vi "Configure IQ Input.vi"(6 "Voltage Level (0.4 V)":dbl=0.4, 7 "I/Q Input Level Method (0: Default)":i32(ring) items=["Default", "Manual", "Measurement"], 8 "error in (no error)":errorcluster, 9 "Auto Attenuation (T: Enable)":bool=TRUE, 10 "Attenuation Level (2 dB)":dbl=2.0, 11 "VISA resource name":refnum<visa-resource-name>) -> (0 "error out":errorcluster, 3 "VISA resource name out":refnum<visa-resource-name>)   [LabVIEW 2012, in "Agilent PSG MXG Series.lvlib"]
doc: "Configures attenuation mode, attenuation level, external I/Q input level and method.\n\n<B>Notes:</B>\n(1) This VI is valid only in N5172B and N5182B."
uses:
  <instrlib>/Agilent PSG MXG Series/Agilent PSG MXG Series.lvlib
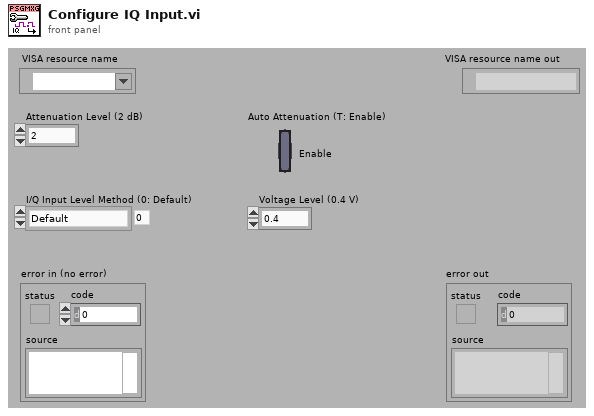
[diagram p1: front panel]
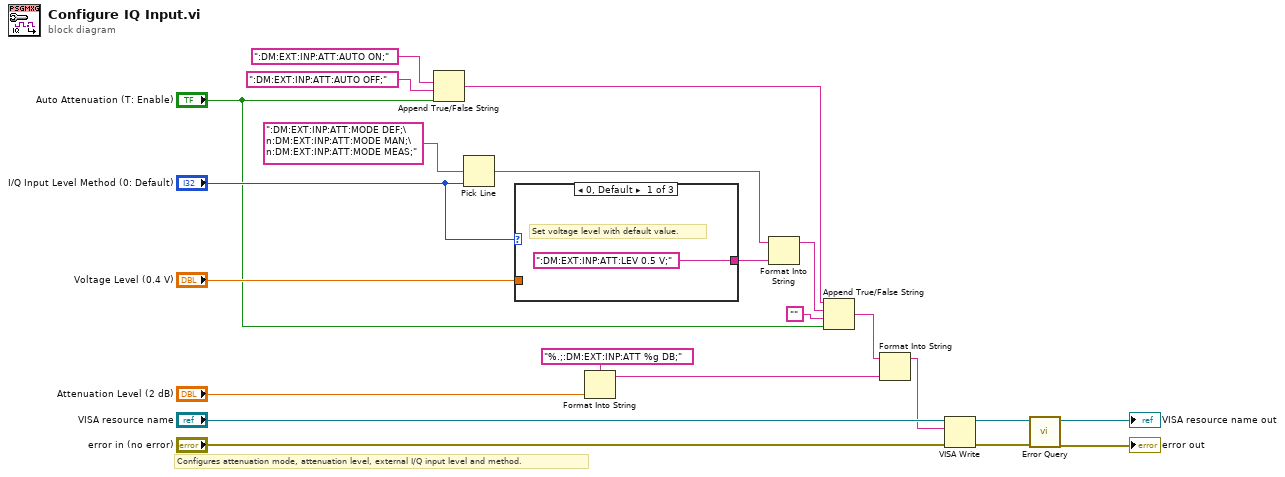
[diagram p0: block diagram]
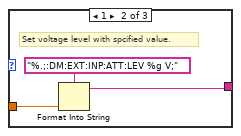
[diagram p2: hidden frame]
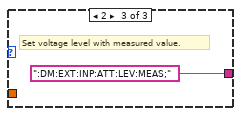
[diagram p3: hidden frame]
diagram:
  # "Configures attenuation mode, attenuation level, external I/Q input level and method."
  n1 = Append True/False String(1:"Auto Attenuation (T: Enable)", 2:":DM:EXT:INP:ATT:AUTO OFF;", 3:":DM:EXT:INP:ATT:AUTO ON;") -> (0:w7:string)  [unwired: 1 out]
  n2 = Pick Line(multi-line string=":DM:EXT:INP:ATT:MODE DEF;\n:DM:EXT:INP:ATT:MODE MAN;\n:DM:EXT:INP:ATT:MODE MEAS;", line index="I/Q Input Level Method (0: Default)") -> (output string=w10:string)  [unwired: 1 out]
  n3 = case shown="0, Default" "I/Q Input Level Method (0: Default)" {
    tunnel: "Voltage Level (0.4 V)" -> [_ w25 _]
    tunnel: [":DM:EXT:INP:ATT:LEV 0.5 V;" w24 ":DM:EXT:INP:ATT:LEV:MEAS;"] -> w9
    frame 0, Default {
      # "Set voltage level with default value."
    }
    frame 1 {
      # "Set voltage level with spcified value."
      n4 = Format Into String(format string="%.;:DM:EXT:INP:ATT:LEV %g V;", w25) -> (resulting string=w24:string)  [unwired: 2 in, 1 out]
    }
    frame 2 {
      # "Set voltage level with measured value."
    }
  }
  n5 = Format Into String(format string="%.;:DM:EXT:INP:ATT %g DB;", "Attenuation Level (2 dB)") -> (resulting string=w2:string)  [unwired: 2 in, 1 out]
  n6 = Format Into String(initial string=w10, w9) -> (resulting string=w6:string)  [unwired: 2 in, 1 out]
  n7 = Append True/False String(1:"Auto Attenuation (T: Enable)", 2:"", 3:w6, 4:w7) -> (0:w3:string)
  n8 = Format Into String(initial string=w3, w2) -> (resulting string=w1:string)  [unwired: 2 in, 1 out]
  n9 = VISA Write(VISA resource name="VISA resource name", write buffer=w1, error in (no error)="error in (no error)") -> (VISA resource name out=w16:refnum<visa-resource-name>, error out=w15:errorcluster)  [unwired: 1 out]
  n10 = call <instrlib>:"Error Query.vi"("error in (no error)"=w15, "VISA resource name"=w16) -> ("error out"=→"error out":errorcluster, "VISA resource name out"=→"VISA resource name out":refnum<visa-resource-name>)  [unwired: 8 out]
